vi "Clear Errors by Codes.vi"(4 "Error Codes\nto Clear (Empty)":i32[](array[numeric]), 5 "error in (no error)":errorcluster) -> (1 "error out":errorcluster)   [LabVIEW 2011]
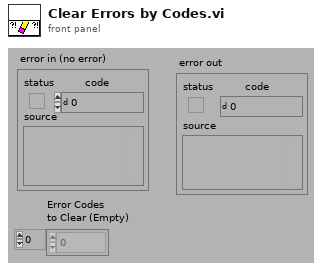
[diagram p1: front panel]
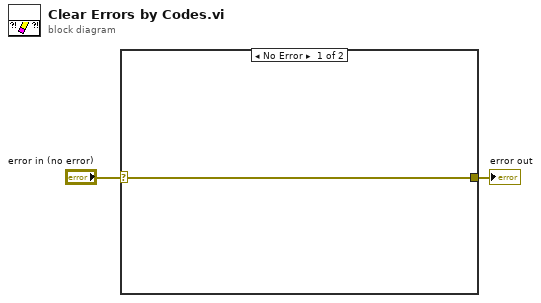
[diagram p0: block diagram]
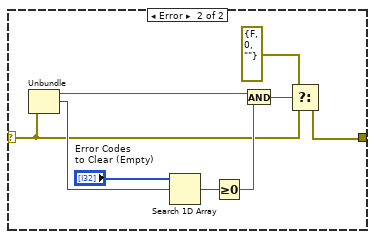
[diagram p2: hidden frame]
diagram:
  n1 = case shown="No Error" "error in (no error)" {
    selector: "error in (no error)" -> [w3 w5]
    tunnel: [w3 w9] -> w1
    frame No Error {
    }
    frame Error {
      n2 = Unbundle(w5) -> ("status"=w12:bool, "code"=w6:i32)  [unwired: 1 out]
      n3 = Search 1D Array(1D array="Error Codes\nto Clear (Empty)", element=w6) -> (index of element=w8:i32)  [unwired: 1 out]
      n4 = Greater Or Equal To 0?(x=w8) -> (x >= 0?=w7:bool)
      n5 = And(x=w12, y=w7) -> (x .and. y?=w11:bool)
      n6 = Select(t=errorcluster {"status"=FALSE, "code"=0, "source"=""} ("error out"), s=w11, f=w5) -> (s? t:f=w9:errorcluster)
    }
  }
  "error out" <- w1
